vi "Abort VIs.vi"(7 "TreeControl in":refnum<vi>, 8 "error in (no error)":errorcluster, 10 "VIs":string[](array[string]), 11 "App":refnum<vi>) -> (0 "error out":errorcluster)   [LabVIEW 2013, in "LVTM.lvlib"]
uses:
  LVTM.lvlib
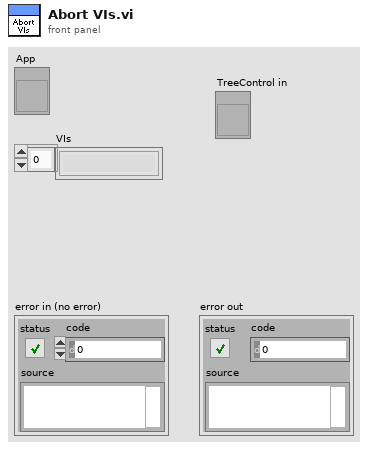
[diagram p1: front panel]
types:
  T1 = enum32{"Bad", "Idle", "Run top level", "Running"}
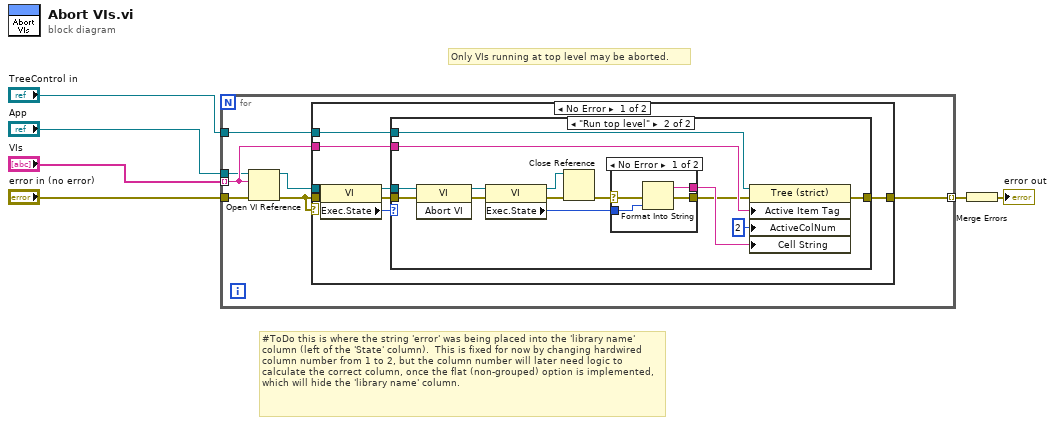
[diagram p0: block diagram]
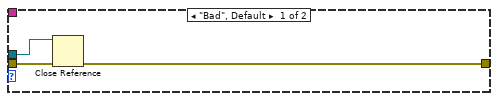
[diagram p2: hidden frame]
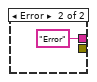
[diagram p3: hidden frame]
diagram:
  # "#ToDo this is where the string 'error' was being placed into the 'library name' column (left of the 'State' column).  This is fixed for now by changing hardwired column number from 1 to 2, but the column number will later need logic to calculate the correct column, once the flat (non-grouped) option is implemented, which will hide the 'library name' column."
  # "Only VIs running at top level may be aborted."
  n1 = for {
    tunnel: [w13] -> w5 mode=indexing
    tunnel: "VIs" -> [w12] mode=indexing
    tunnel: "App" -> [w11]
    tunnel: "error in (no error)" -> [w10]
    tunnel: "TreeControl in" -> [w7]
    n2 = Open VI Reference(application reference (local)=w11, vi path=w12, error in (no error)=w10) -> (vi reference=w9:refnum<vi>, error out=w8:errorcluster)  [unwired: 3 out]
    n3 = case shown="No Error" w8 {
      tunnel: [w21 _] -> w13
      tunnel: w12 -> [w20 _]
      tunnel: w8 -> [w19 _]
      tunnel: w9 -> [w17 _]
      tunnel: w7 -> [w14 _]
      frame No Error {
        n4 = property class="VI"(reference=w17, error in=w19) -> (reference out=w16:refnum<vi>, error out=w18:errorcluster, "Exec.State"=w15:T1)
        n5 = case shown="\"Run top level\"" w15 {
          tunnel: [w22 w35] -> w21
          tunnel: w20 -> [_ w33]
          tunnel: w18 -> [w24 w28]
          tunnel: w16 -> [w23 w27]
          tunnel: w14 -> [_ w25]
          frame "Bad", Default {
            n6 = Close Reference(reference=w23, error in (no error)=w24) -> (error out=w22:errorcluster)
          }
          frame "Run top level" {
            n7 = invoke class="VI" method="Abort VI"(reference=w27, error in=w28) -> (reference out=w37:refnum<vi>, error out=w29:errorcluster)  [unwired: 1 in, 1 out]
            n8 = property class="VI"(reference=w37, error in=w29) -> (reference out=w36:refnum<vi>, error out=w31:errorcluster, "Exec.State"=w38:T1)
            n9 = Close Reference(reference=w36, error in (no error)=w31) -> (error out=w26:errorcluster)
            n10 = case shown="No Error" w26 {
              selector: w26 -> [w39 _]
              tunnel: w38 -> [w42 _]
              tunnel: [w41 "Error"] -> w34
              tunnel: [w40 _] -> w30
              frame No Error {
                n11 = Format Into String(error in=w39, w42) -> (resulting string=w41:string, error out=w40:errorcluster)  [unwired: 2 in]
              }
              frame Error {
              }
            }
            n12 = property on="Property Node" class="Tree (strict)"(reference=w25, error in=w30, "Active Item Tag"=w33, "ActiveColNum"=2 ("Active Cell:Active Column Number"), "Cell String"=w34) -> (error out=w35:errorcluster)  [unwired: 1 out]
          }
        }
      }
      frame Error {
        # "This VI is no longer in the memory"
      }
    }
  }
  n13 = Merge Errors(w5) -> (→"error out":errorcluster)
